vi "Interfaz grafica - corriente.vi"() -> ()   [LabVIEW 2024]
uses:
  160620 Optotune Lens Driver 4 Labview package/Hello Optotune Lens (30.06.2015)/Calibration.ctl
  <vilib>/Utility/file.llb/Read Delimited Spreadsheet (string).vi
  <vilib>/Instr/_visa.llb/VISA Configure Serial Port (Instr).vi
  <vilib>/Utility/file.llb/Write Delimited Spreadsheet (string).vi
panel:
  in  "Numeric WL control":i32
  in  "stop 6":bool
  in  "stop 5":bool
  in  "stop 4":bool
  in  "stop 3":bool
  in  "stop 2":bool
  in  "stop":bool
  out "Array 4":string[](array[string])
  out "Array 3":string[](array[string])
  out "Array 2":string[](array[string])
  out "Array":string[](array[string])
  out "Nombre 2":string
  in  "Restablecer Iniciales":bool
  in  "Incremento":dbl=0.1 format="%#_13g"
  out "Potencia derecho":dbl
  out "error out 4":errorcluster
  out "error out 3":errorcluster
  out "error out 2":errorcluster
  out "VISA resource name out":string
  in  "Tab Control 2":T1(tab)
  in  "Potencia inicial lente derecho":dbl(slide) scale=-3.0..3.0
  in  "Potencia inicial lente izquierdo":dbl(slide) scale=-3.0..3.0
  in  "VISA resource name":string="COM11"
  in  "VISA resource name 2":string="COM10"
  out "DPT INICIALES D":dbl
  out "DPT INICIALES I":dbl
  out "Potencia izquierdo":dbl
  in  "error in (no error) 5":errorcluster
  in  "error in (no error) 4":errorcluster
  in  "error in (no error) 3":errorcluster
  in  "error in (no error) 2":errorcluster
  in  "Calibration 4":T2={"Max Current A"=293.0, "Max Current B"=293.0, "UCL A"=300.0, "UCL B"=300.0, "LCL A"=0.0, "LCL B"=0.0} {"Max Current A" format="%#_g mA"; "Max Current B" format="%#_g mA"; "UCL A" format="%#_g mA"; "LCL A" format="%#_g mA"; "UCL B" format="%#_g mA"; "LCL B" format="%#_g mA"}
  out "ID 2":u16
  out "VISA resource name out 2":string
  out "Calibration 3":T2 {"Max Current A" format="%#_g mA"; "Max Current B" format="%#_g mA"; "UCL A" format="%#_g mA"; "LCL A" format="%#_g mA"; "UCL B" format="%#_g mA"; "LCL B" format="%#_g mA"}
  out "OK 2":bool
  out "Data 2":string
  out "Command to Port 2":string
  in  "Calibration":T2={"Max Current A"=293.0, "Max Current B"=293.0, "UCL A"=300.0, "UCL B"=300.0, "LCL A"=0.0, "LCL B"=0.0} {"Max Current A" format="%#_g mA"; "Max Current B" format="%#_g mA"; "UCL A" format="%#_g mA"; "LCL A" format="%#_g mA"; "UCL B" format="%#_g mA"; "LCL B" format="%#_g mA"}
  out "ID":u16
  out "Calibration 2":T2 {"Max Current A" format="%#_g mA"; "Max Current B" format="%#_g mA"; "UCL A" format="%#_g mA"; "LCL A" format="%#_g mA"; "UCL B" format="%#_g mA"; "LCL B" format="%#_g mA"}
  out "OK":bool
  out "Data":string
  out "Command to Port":string
  in  "DPT dif.":dbl
  out "error out":errorcluster
  in  "error in (no error)":errorcluster
  out "T button?":bool
  in  "Elegir menu Exp":bool
  in  "Elegir menu":bool
  out "path":path
  in  "Iniciar experimento":bool
  out "Enfermedad visual":string
  out "Edad":string
  out "Nombre":string
  out "Cedula":string
  in  "Carpeta":path=path "C:/Users/TGM1603/Documents/LabVIEW Data/Experimentos electrodos"
  in  "?":bool
  in  "Menu Principal":u16(ring) items=["Visualizacion general ", "Llevar a cabo un experimento", "Ajustar potencia inicial lentes"]
  in  "Menu experimentos":u16(ring) items=["Experimento 1", "Experimento 2", "Experimento 3", "Experimento 4"]
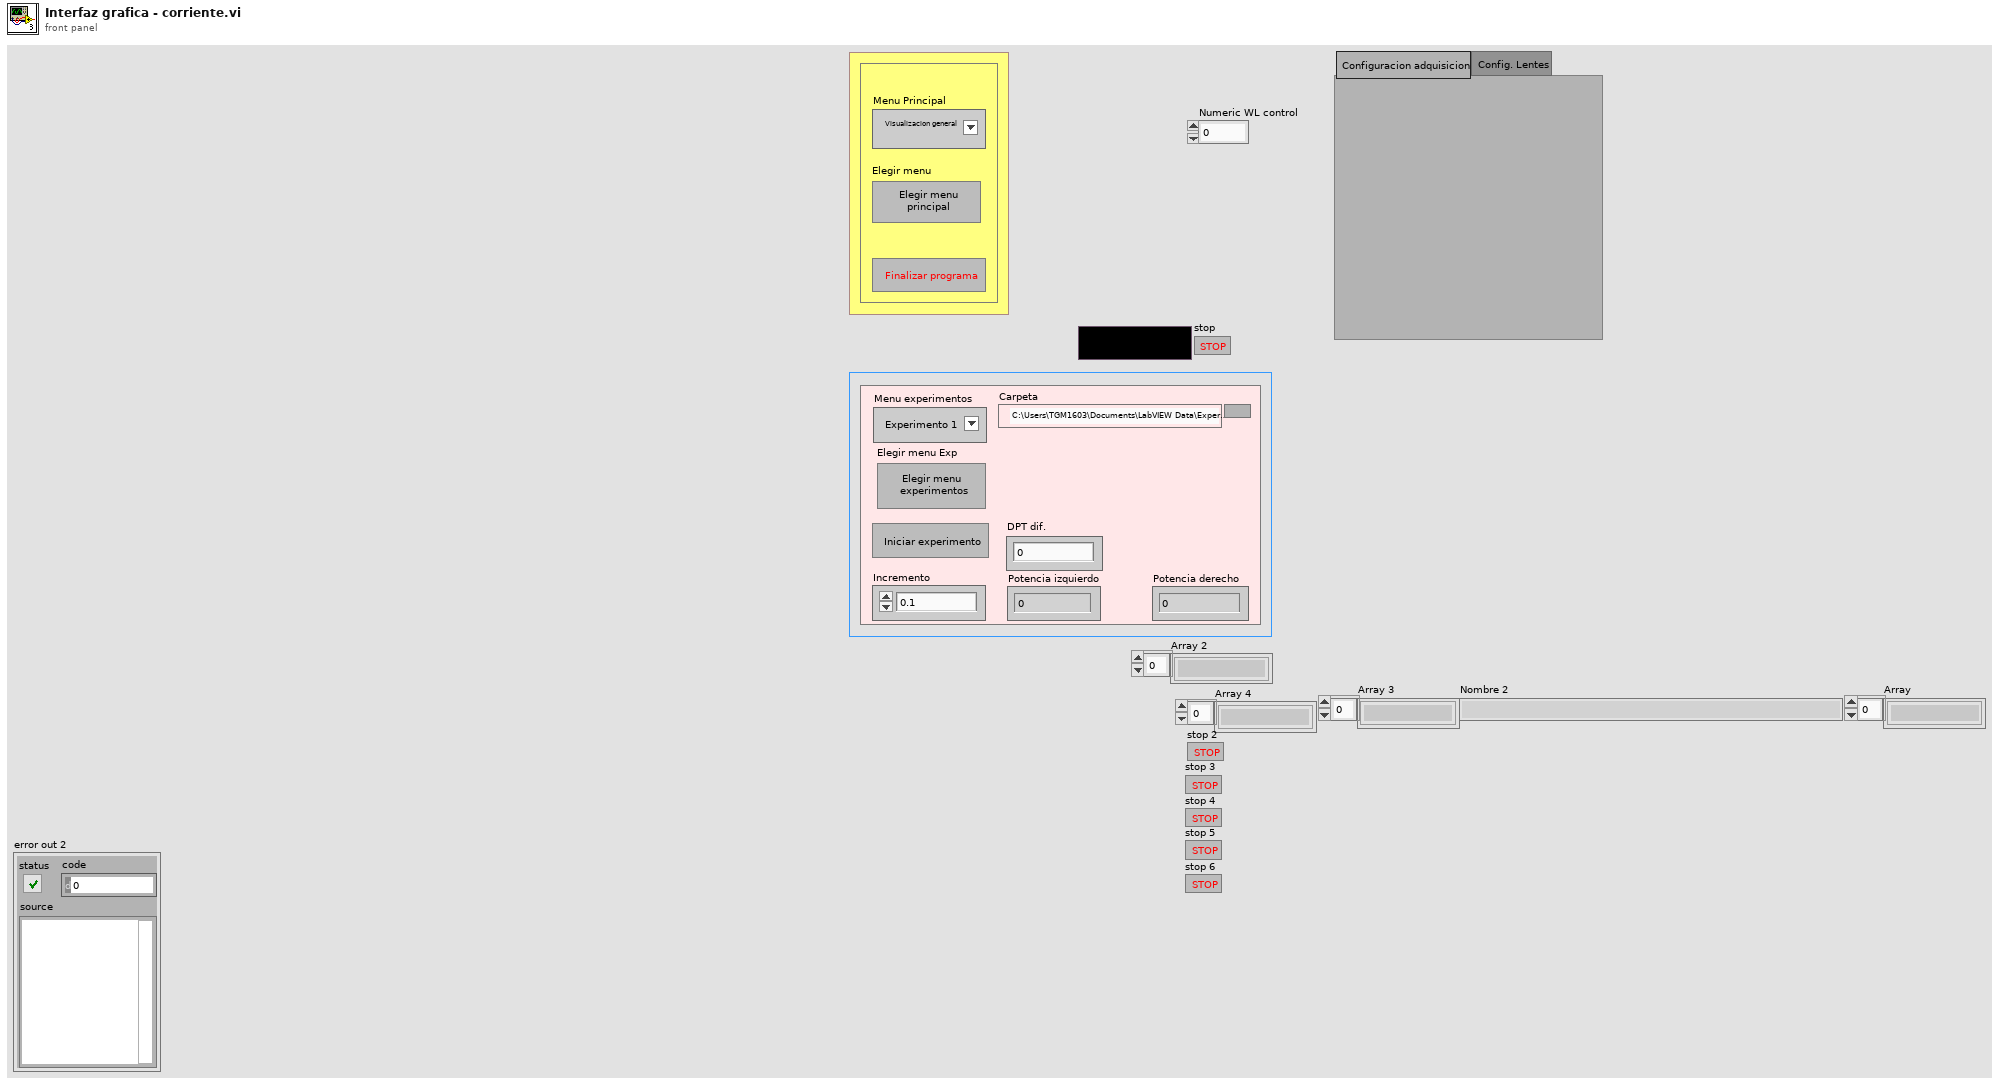
[diagram p1: front panel]
types:
  T1 = enum32{"Configuracion adquisicion", "Config. Lentes"}
  T2 = typedef "Calibration.ctl" = cluster{"Max Current A":dbl, "Max Current B":dbl, "UCL A":dbl, "UCL B":dbl, "LCL A":dbl, "LCL B":dbl}
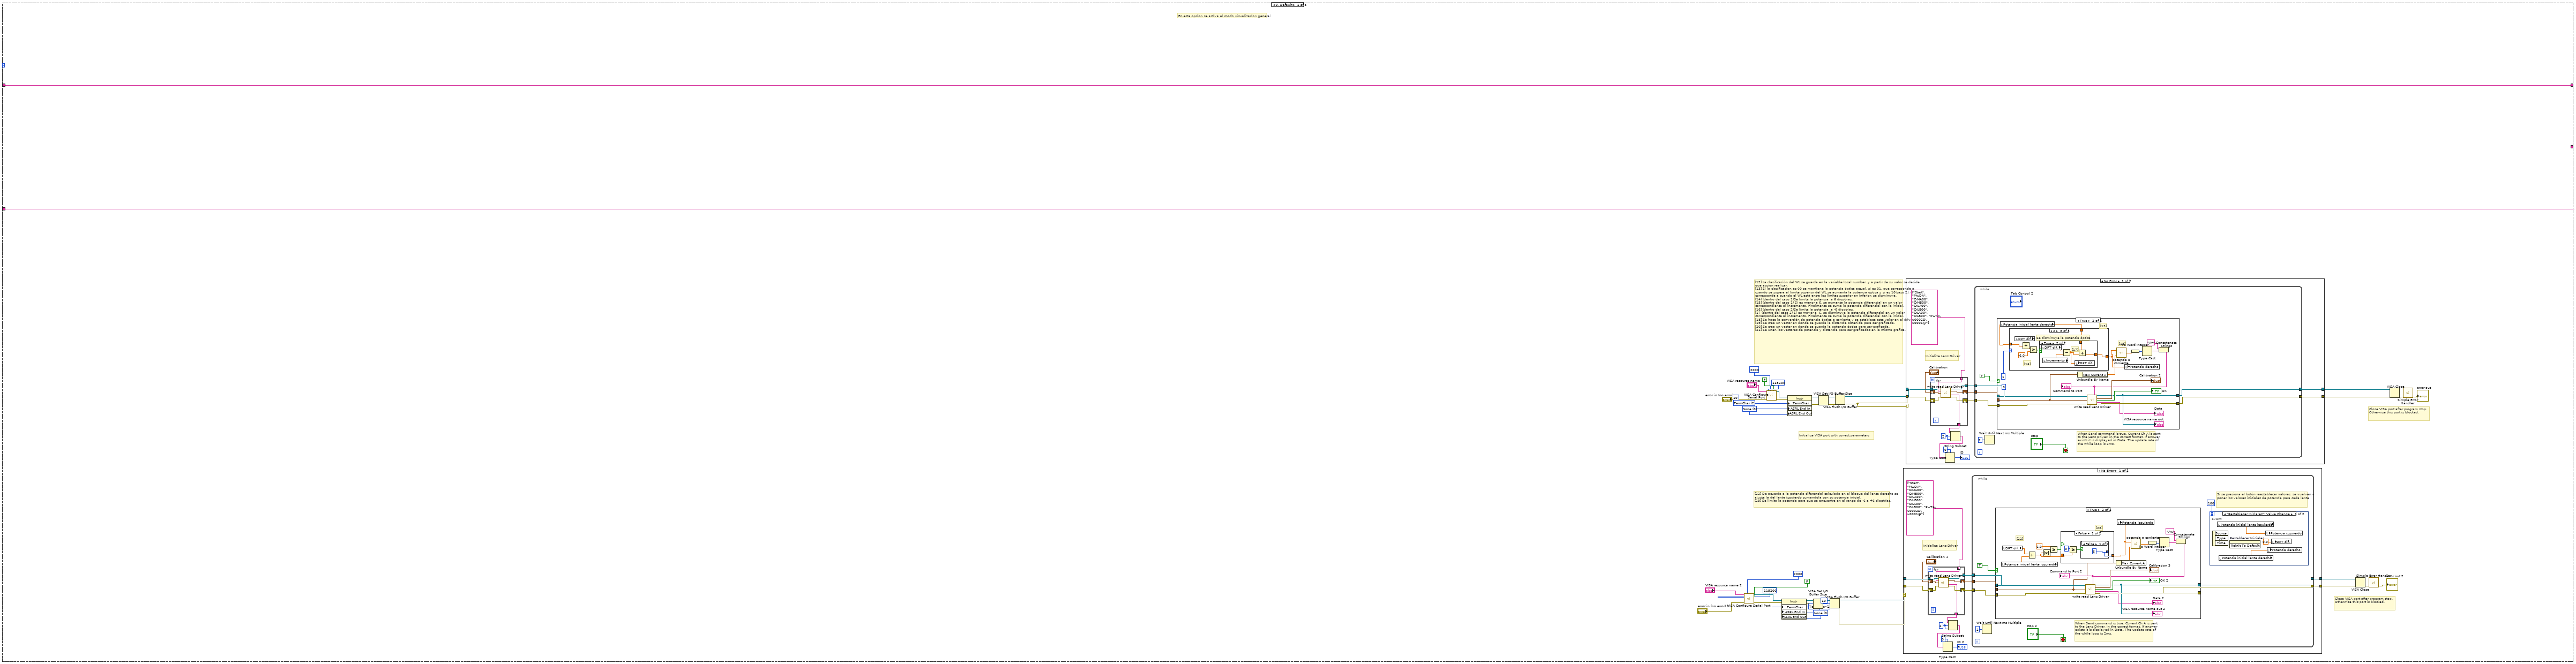
[diagram p2: hidden frame]
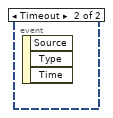
[diagram p3: hidden frame]
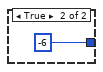
[diagram p5: hidden frame]
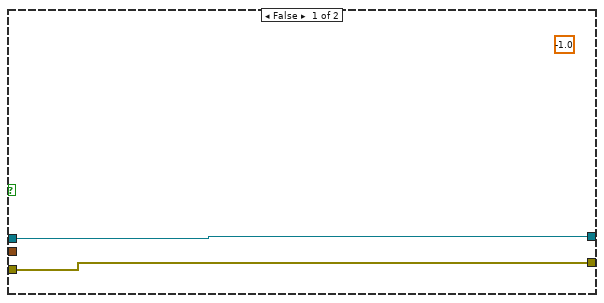
[diagram p8: hidden frame]
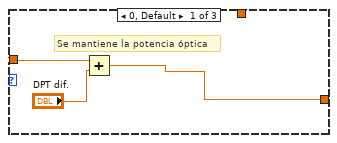
[diagram p9: hidden frame]
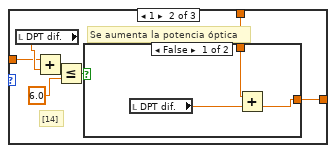
[diagram p10: hidden frame]
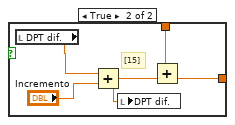
[diagram p11: hidden frame]
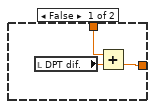
[diagram p12: hidden frame]
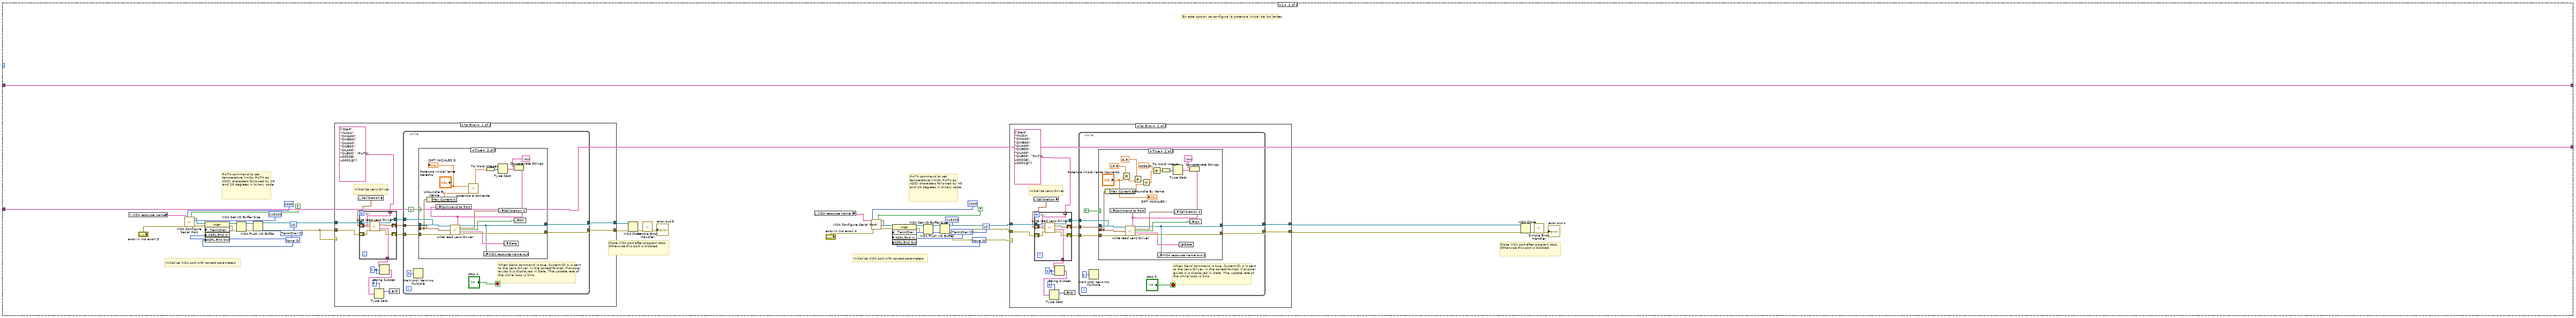
[diagram p14: hidden frame]
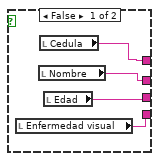
[diagram p19: hidden frame]
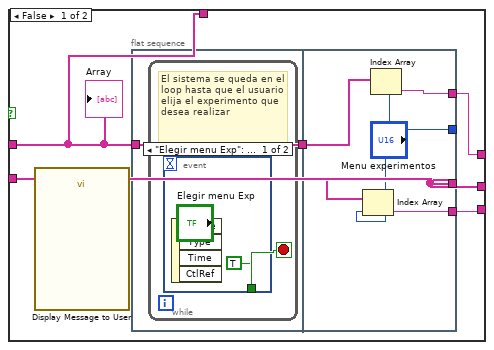
[diagram p20: hidden frame]
diagram:
  n1 = flat-sequence {
    tunnel: [w9] -> w2
    tunnel: [w6] -> w1
    tunnel: w2 -> [w13]
    tunnel: w1 -> [w14]
    frame #0 {
      # "Se inicializan los valores\nde potencia óptica y WL"
      # "Crea la cola que va a guardar los valores de la sumatoria que calcula el waveform length así como determina la cantidad de valores que se van a sumar(tamaño de la ventana)"
      # "Se obtiene los elementos de la columna 1 que corresponde a  la descripcion de los experimentos"
      # "Se obtiene los elementos de la columna 0 que corresponde al nombre de los experimentos"
      # "Se guarda los experimentos en el menu\n para que el usuario pueda elegir cual \nrealizar"
      # "Se cargan los experimentos  guardados"
      n2 = call-poly <vilib>:"Read Delimited Spreadsheet.vi"("file path (dialog if empty)"=path "C:/Users/willi/GITHUB/TG/Interfaz grafica -LabVIEW/Try 1/TG Juan Diego/Documentos de Labview/Experimentos_realizados") -> ("all rows"=w10:string[][])  [unwired: 9 in, 5 out]
      n3 = Transpose 2D Array(2D array=w10) -> (transposed array=w7:string[][])
      n4 = Index Array(array=w7, index (row)=1) -> (element=w6:string[])  [unwired: 1 in]
      n5 = Index Array(array=w7, index (row)=0) -> (element=w9:string[])  [unwired: 1 in]
      n6 = property on="Menu experimentos" class="Ring (strict)"("Strings []"=w9) -> ()  [unwired: 2 in, 2 out]
      n7 = local write "DPT INICIALES D"(0.0 ("DPT INIT.1")) -> ()
      n8 = local write "DPT INICIALES I"(0.0 ("DPT INIT.2")) -> ()
      n9 = local write "DPT dif."(0.0 ("WL")) -> ()
    }
    frame #1 {
      n10 = while {
        shift-right: [w19] -> _
        shift-left: w13 -> [w20]
        shift-right: [w17] -> _
        shift-left: w14 -> [w18]
        stop <- w16 stop-if-true
        n11 = event shown="[0] \"Elegir menu\": Value Change" {
          selector: _ -> [_ _]
          dyn-events: _ -> [_ _]
          timeout: 10 -> [_ _]
          tunnel: w20 -> [w25 w718]
          tunnel: [w24 w718] -> w19
          tunnel: w18 -> [w23 w717]
          tunnel: [w22 w717] -> w17
          tunnel: [_ "?"] -> w16
          event "Elegir menu": Value Change {
            n12 = event-data() -> ()  [unwired: 1 in, 6 out]
            n13 = case shown="1" "Menu Principal" {
              tunnel: w25 -> [w67 w259 w372]
              tunnel: [w67 w259 w371] -> w24
              tunnel: w23 -> [w66 w258 w369]
              tunnel: [w66 w258 w368] -> w22
              frame 0, Default {
                w41 = u16 0 items=["None", "Last Bit", "TermChar", "Break"] ("Serial Settings:End Mode for Writes")
                w40 = u16 2 items=["None", "Last Bit", "TermChar"] ("Serial Settings:End Mode for Reads")
                w56 = u16 0 items=["None", "Last Bit", "TermChar", "Break"] ("Serial Settings:End Mode for Writes")
                w57 = u16 2 items=["None", "Last Bit", "TermChar"] ("Serial Settings:End Mode for Reads")
                # "[22] De acuerda a la potencia diferencial calculada en el bloque del lente derecho se ajusta la del lente izquierdo sumandola con su potencia inicial.\n[23] Se limita la potencia para que se encuentre en el rango de -6 a +6 dioptrías."
                # "[12] La clasificación del WL se guarda en la variable local number, y a partir de su valor se decide que accion realizar.\n[13] Si la clasificacion es 00 se mantiene la potencia óptica actual, si es 01, que corresponde a cuando se supera el limite superior del WL,se aumenta la potencia óptica y si es 10(caso 2), que corresponde a cuando el WL está entre los limites superior en inferior, se disminuye. \n[14] (dentro del caso 1)Se limita la potencia  a 6 dioptrías. \n[15] (dentro del caso 1) Si es menor a 6, se aumenta la potencia diferencial en un valor correspondiente al incremento. Finalmente se suma la potencia diferencial con la inicial.\n[16] (dentro del caso 2)Se limita la potencia  a -6 dioptrías.\n[17 (dentro del caso 2) Si es mayor a -6, se disminuye la potencia diferencial en un valor correspondiente al incremento. Finalmente se suma la potencia diferencial con la inicial.\n[18] Se hace la conversión de potencia óptica a corriente y se establece este valor en el driver.\n[19] Se crea un vector en donde se guarda la distancia obtenida para ser graficada.\n[20] Se crea un vector en donde se guarda la potencia óptica para ser graficada.\n[21] Se unen los vectores de potencia y distancia para ser graficados en la misma grafica."
                # "En esta opcion se activa el modo visualizacion general"
                # "Close VISA port after program stop. Otherwise this port is blocked."
                # "Close VISA port after program stop. Otherwise this port is blocked."
                # "Initialize VISA port with correct parameters"
                n14 = call-poly "VISA Configure Serial Port"("VISA resource name"="VISA resource name 2", "timeout (10sec)"=u32 2000, "Enable Termination\nChar (T)"=FALSE ("Enable Termination\nChar (T)"), "baud rate (9600)"=u32 115200, "error in (no error)"="error in (no error) 2") -> ("VISA resource name out"=w36:refnum<visa-resource-name>, "error out"=w38:errorcluster)  [unwired: 9 in]
                n15 = call-poly "VISA Configure Serial Port"("VISA resource name"="VISA resource name", "timeout (10sec)"=u32 2000, "Enable Termination\nChar (T)"=FALSE ("Enable Termination\nChar (T)"), "baud rate (9600)"=u32 115200, "error in (no error)"="error in (no error)") -> ("VISA resource name out"=w61:refnum<visa-resource-name>, "error out"=w59:errorcluster)  [unwired: 9 in]
                n16 = property class="Instr"(reference=w36, error in=w38, "TermChar"=u8 10 ("Message Based Settings:Termination Character"), "ASRL End In"=w40, "ASRL End Out"=w41) -> (reference out=w37:refnum<visa-resource-name>, error out=w39:errorcluster)
                n17 = property class="Instr"(reference=w61, error in=w59, "TermChar"=u8 10 ("Message Based Settings:Termination Character"), "ASRL End In"=w57, "ASRL End Out"=w56) -> (reference out=w60:refnum<visa-resource-name>, error out=w58:errorcluster)
                n18 = VISA Set I/O Buffer Size(VISA resource name=w37, error in (no error)=w39) -> (VISA resource name out=w44:refnum<visa-resource-name>, error out=w45:errorcluster)  [unwired: 2 in]
                n19 = VISA Set I/O Buffer Size(VISA resource name=w60, error in (no error)=w58) -> (VISA resource name out=w53:refnum<visa-resource-name>, error out=w52:errorcluster)  [unwired: 2 in]
                n20 = VISA Flush I/O Buffer(VISA resource name=w44, error in (no error)=w45) -> (VISA resource name out=w30:refnum<visa-resource-name>, error out=w31:errorcluster)  [unwired: 1 in]
                n21 = VISA Flush I/O Buffer(VISA resource name=w53, error in (no error)=w52) -> (VISA resource name out=w51:refnum<visa-resource-name>, error out=w46:errorcluster)  [unwired: 1 in]
                n22 = case shown="No Error" w31 {
                  tunnel: w31 -> [w81 w132]
                  tunnel: w30 -> [w80 w133]
                  tunnel: [w79 w132] -> w26
                  tunnel: [w78 w133] -> w27
                  frame No Error {
                    w76 = 2 ("length (rest)")
                    # "Initialize Lens Driver"
                    n23 = for {
                      tunnel: w80 -> [w130]
                      tunnel: [w127] -> w70
                      tunnel: string[] ["Start", "MwDA", "CrMA00", "CrMB00", "CrUA00", "CrUB00", "CrLA00", "CrLB00", "PwTA\u0002Ð\u0001@"] -> [w125] mode=indexing
                      tunnel: [w124] -> w69
                      shift-right: [w128] -> w71
                      shift-left: "Calibration 4" -> [w129]
                      shift-right: [w126] -> w72
                      shift-left: w81 -> [w131]
                      n24 = call "write read Lens Driver.vi"("VISA resource name"=w130, "command"=w125, "Calibration"=w129, "error in (no error)"=w131) -> ("VISA resource name out"=w127:refnum<visa-resource-name>, "Calibration 2"=w128:T2, "Data"=w124:string, "error out"=w126:errorcluster)  [unwired: 4 in, 4 out]
                    }
                    n25 = String Subset(string=w69, offset (0)=w76, length (rest)=w76) -> (substring=w74:string)
                    n26 = Type Cast(type=u16 0 ("length (rest)"), x=w74) -> (*(type *) &x=→"ID 2":u16)
                    n27 = while {
                      tunnel: [w84] -> w79
                      tunnel: [w85] -> w78
                      tunnel: w72 -> [w90]
                      tunnel: w71 -> [w89]
                      tunnel: w70 -> [w88]
                      stop <- "stop 2" stop-if-true
                      # "Si se presiona el botón reestablecer valores, se vuelven a poner los valores iniciales de potencia para cada lente"
                      # "When Send command is true, Current Ch A is sent to the Lens Driver, in the correct format. If answer exists it is displayed in Data. The update rate of the while loop is 2ms."
                      n28 = Wait Until Next ms Multiple(millisecond multiple=u32 2) -> ()  [unwired: 1 out]
                      n29 = case shown="True" TRUE ("Send command") {
                        tunnel: [w95 w116] -> w84
                        tunnel: w90 -> [w95 w115]
                        tunnel: w89 -> [_ w97]
                        tunnel: w88 -> [w94 w114]
                        tunnel: [w94 w111] -> w85
                        frame False {
                        }
                        frame True {
                          # "[23]"
                          # "[22]"
                          n30 = local read "Potencia inicial lente izquierdo"() -> (w105:dbl)
                          n31 = local read "DPT dif."() -> (w106:dbl)
                          n32 = Add(x=w106, y=w105) -> (x+y=w101:dbl)
                          n33 = Absolute Value(x=w101) -> (abs(x)=w103:dbl)
                          n34 = Greater Or Equal?(x=6.0, y=w103) -> (x >= y?=w104:bool)
                          n35 = case shown="False" w104 {
                            tunnel: w101 -> [w119 w123]
                            tunnel: [w117 w123] -> w99
                            frame False {
                              n36 = Greater Or Equal?(x=u16 0, y=w119) -> (x >= y?=w120:bool)
                              n37 = case shown="False" w120 {
                                tunnel: [i16 6 ("x") i16 -6 ("x")] -> w117
                                frame False {
                                }
                                frame True {
                                }
                              }
                            }
                            frame True {
                            }
                          }
                          n38 = Unbundle By Name(w97) -> ("Max Current A"=w98:dbl)
                          n39 = local write "Potencia izquierdo"(w99) -> ()
                          n40 = call "potencia a corriente.vi"("Max current A"=w98, "Potencia"=w99) -> ("Corriente"=w100:dbl)
                          n41 = To Word Integer(number=w100) -> (16bit integer=w109:i16)
                          n42 = Type Cast(x=w109) -> (*(type *) &x=w108:string)  [unwired: 1 in]
                          n43 = Concatenate Strings("Aw", w108) -> (w107:string)
                          "Command to Port 2" <- w107
                          n44 = call "write read Lens Driver.vi"("VISA resource name"=w114, "command"=w107, "Calibration"=w97, "error in (no error)"=w115) -> ("VISA resource name out"=w111:refnum<visa-resource-name>, "Calibration 2"=→"Calibration 3":T2, "OK"=→"OK 2":bool, "Data"=→"Data 2":string, "error out"=w116:errorcluster)  [unwired: 4 in, 3 out]
                          "VISA resource name out 2" <- w111
                        }
                      }
                      n45 = event shown="[0] \"Restablecer Iniciales\": Value Change" {
                        selector: _ -> [_ _]
                        dyn-events: _ -> [_ _]
                        timeout: 100 -> [_ _]
                        event "Restablecer Iniciales": Value Change {
                          n46 = event-data() -> ()  [unwired: 1 in, 3 out]
                          n47 = local read "Potencia inicial lente izquierdo"() -> (w91:dbl)
                          n48 = local read "Potencia inicial lente derecho"() -> (w92:dbl)
                          n49 = invoke on="Restablecer Iniciales" class="Bool" method="Reinit To Default"() -> ()  [unwired: 3 in, 3 out]
                          n50 = local write "Potencia izquierdo"(w91) -> ()
                          n51 = local write "Potencia derecho"(w92) -> ()
                          n52 = local write "DPT dif."(0.0 ("DPT dif.")) -> ()
                        }
                        event Timeout {
                          n53 = event-data() -> ()  [unwired: 1 in, 3 out]
                        }
                      }
                    }
                  }
                  frame Error {
                  }
                }
                n54 = case shown="No Error" w46 {
                  tunnel: w46 -> [w147 w216]
                  tunnel: w51 -> [w146 w217]
                  tunnel: [w145 w216] -> w49
                  tunnel: [w144 w217] -> w47
                  frame No Error {
                    w142 = 2 ("length (rest)")
                    # "Initialize Lens Driver"
                    n55 = for {
                      tunnel: w146 -> [w214]
                      tunnel: [w211] -> w136
                      tunnel: string[] ["Start", "MwDA", "CrMA00", "CrMB00", "CrUA00", "CrUB00", "CrLA00", "CrLB00", "PwTA\u0002Ð\u0001@"] -> [w209] mode=indexing
                      tunnel: [w208] -> w135
                      shift-right: [w212] -> w137
                      shift-left: "Calibration" -> [w213]
                      shift-right: [w210] -> w138
                      shift-left: w147 -> [w215]
                      n56 = call "write read Lens Driver.vi"("VISA resource name"=w214, "command"=w209, "Calibration"=w213, "error in (no error)"=w215) -> ("VISA resource name out"=w211:refnum<visa-resource-name>, "Calibration 2"=w212:T2, "Data"=w208:string, "error out"=w210:errorcluster)  [unwired: 4 in, 4 out]
                    }
                    n57 = String Subset(string=w135, offset (0)=w142, length (rest)=w142) -> (substring=w140:string)
                    n58 = Type Cast(type=u16 0 ("length (rest)"), x=w140) -> (*(type *) &x=→"ID":u16)
                    n59 = while {
                      tunnel: [w149] -> w145
                      tunnel: [w150] -> w144
                      tunnel: w138 -> [w155]
                      tunnel: w137 -> [w154]
                      tunnel: w136 -> [w153]
                      stop <- "stop" stop-if-true
                      # "When Send command is true, Current Ch A is sent to the Lens Driver, in the correct format. If answer exists it is displayed in Data. The update rate of the while loop is 2ms."
                      n60 = Wait Until Next ms Multiple(millisecond multiple=u32 2) -> ()  [unwired: 1 out]
                      n61 = case shown="True" TRUE ("Send command") {
                        tunnel: [w157 w174] -> w149
                        tunnel: w155 -> [w157 w173]
                        tunnel: w154 -> [_ w161]
                        tunnel: w153 -> [w156 w172]
                        tunnel: [w156 w169] -> w150
                        frame False {
                          (unwired) -1.0 ("DPT")
                        }
                        frame True {
                          (unwired) 0
                          # "[18]"
                          # "[13]"
                          n62 = local read "Potencia inicial lente derecho"() -> (w164:dbl)
                          n63 = case shown="2" 1 {
                            tunnel: [w176 w184 w199] -> w163
                            tunnel: w164 -> [w177 w179 w194]
                            tunnel: w164 -> [_ w178 w193]
                            frame 0, Default {
                              # "Se mantiene la potencia óptica"
                              n64 = Add(x=w177, y="DPT dif.") -> (x+y=w176:dbl)
                            }
                            frame 1 {
                              # "[14]"
                              # "Se aumenta la potencia óptica"
                              n65 = local read "DPT dif."() -> (w180:dbl)
                              n66 = Add(x=w179, y=w180) -> (x+y=w181:dbl)
                              n67 = Less Or Equal?(x=w181, y=6.0) -> (x <= y?=w183:bool)
                              n68 = case shown="False" w183 {
                                tunnel: [w186 w189] -> w184
                                tunnel: w178 -> [w185 w188]
                                frame False {
                                n69 = local read "DPT dif."() -> (w187:dbl)
                                n70 = Add(x=w185, y=w187) -> (x+y=w186:dbl)
                                }
                                frame True {
                                # "[15]"
                                n71 = local read "DPT dif."() -> (w190:dbl)
                                n72 = Add(x=w190, y="Incremento") -> (x+y=w191:dbl)
                                n73 = local write "DPT dif."(w191) -> ()
                                n74 = Add(x=w188, y=w191) -> (x+y=w189:dbl)
                                }
                              }
                            }
                            frame 2 {
                              # "[16]"
                              # "Se disminuye la potencia óptica"
                              n75 = local read "DPT dif."() -> (w198:dbl)
                              n76 = Add(x=w198, y=w194) -> (x+y=w195:dbl)
                              n77 = Greater Or Equal?(x=w195, y=-6.0) -> (x >= y?=w196:bool)
                              n78 = case shown="True" w196 {
                                tunnel: [w201 w205] -> w199
                                tunnel: w193 -> [w200 w204]
                                frame False {
                                n79 = local read "DPT dif."() -> (w202:dbl)
                                n80 = Add(x=w200, y=w202) -> (x+y=w201:dbl)
                                }
                                frame True {
                                # "[17]"
                                n81 = local read "DPT dif."() -> (w207:dbl)
                                n82 = local read "Incremento"() -> (w203:dbl)
                                n83 = Subtract(x=w207, y=w203) -> (x-y=w206:dbl)
                                n84 = local write "DPT dif."(w206) -> ()
                                n85 = Add(x=w204, y=w206) -> (x+y=w205:dbl)
                                }
                              }
                            }
                          }
                          n86 = Unbundle By Name(w161) -> ("Max Current A"=w160:dbl)
                          n87 = call "potencia a corriente.vi"("Max current A"=w160, "Potencia"=w163) -> ("Corriente"=w162:dbl)
                          n88 = local write "Potencia derecho"(w163) -> ()
                          n89 = To Word Integer(number=w162) -> (16bit integer=w167:i16)
                          n90 = Type Cast(x=w167) -> (*(type *) &x=w166:string)  [unwired: 1 in]
                          n91 = Concatenate Strings("Aw", w166) -> (w165:string)
                          "Command to Port" <- w165
                          n92 = call "write read Lens Driver.vi"("VISA resource name"=w172, "command"=w165, "Calibration"=w161, "error in (no error)"=w173) -> ("VISA resource name out"=w169:refnum<visa-resource-name>, "Calibration 2"=→"Calibration 2":T2, "OK"=→"OK":bool, "Data"=→"Data":string, "error out"=w174:errorcluster)  [unwired: 4 in, 3 out]
                          "VISA resource name out" <- w169
                        }
                      }
                    }
                  }
                  frame Error {
                  }
                }
                n93 = VISA Close(VISA resource name=w27, error in (no error)=w26) -> (error out=w28:errorcluster)
                n94 = call <vilib>:"Simple Error Handler.vi"("error in (no error)"=w28) -> ("error out"=→"error out 2":errorcluster)  [unwired: 4 in, 4 out]
                n95 = VISA Close(VISA resource name=w47, error in (no error)=w49) -> (error out=w50:errorcluster)
                n96 = call <vilib>:"Simple Error Handler.vi"("error in (no error)"=w50) -> ("error out"=→"error out":errorcluster)  [unwired: 4 in, 4 out]
              }
              frame 2 {
                w238 = u16 0 items=["None", "Last Bit", "TermChar", "Break"] ("Serial Settings:End Mode for Writes")
                w237 = u16 2 items=["None", "Last Bit", "TermChar"] ("Serial Settings:End Mode for Reads")
                w251 = u16 0 items=["None", "Last Bit", "TermChar", "Break"] ("Serial Settings:End Mode for Writes")
                w250 = u16 2 items=["None", "Last Bit", "TermChar"] ("Serial Settings:End Mode for Reads")
                # "En esta opcion se configura la potencia inicial de los lentes"
                # "Close VISA port after program stop. Otherwise this port is blocked."
                # "Close VISA port after program stop. Otherwise this port is blocked."
                # "PwTA command to set temperature limits: PwTA as ASCII characters followed by 45 and 20 degrees in binary code."
                # "Initialize VISA port with correct parameters"
                # "PwTA command to set temperature limits: PwTA as ASCII characters followed by 45 and 20 degrees in binary code."
                # "Initialize VISA port with correct parameters"
                n97 = local read "VISA resource name"() -> (w228:string)
                n98 = call-poly "VISA Configure Serial Port"("VISA resource name"=w228, "timeout (10sec)"=u32 2000, "Enable Termination\nChar (T)"=FALSE ("Enable Termination\nChar (T)"), "baud rate (9600)"=u32 115200, "error in (no error)"="error in (no error) 3") -> ("VISA resource name out"=w233:refnum<visa-resource-name>, "error out"=w235:errorcluster)  [unwired: 9 in]
                n99 = property class="Instr"(reference=w233, error in=w235, "TermChar"=u8 10 ("Message Based Settings:Termination Character"), "ASRL End In"=w237, "ASRL End Out"=w238) -> (reference out=w234:refnum<visa-resource-name>, error out=w236:errorcluster)
                n100 = VISA Set I/O Buffer Size(VISA resource name=w234, error in (no error)=w236) -> (VISA resource name out=w240:refnum<visa-resource-name>, error out=w241:errorcluster)  [unwired: 2 in]
                n101 = VISA Flush I/O Buffer(VISA resource name=w240, error in (no error)=w241) -> (VISA resource name out=w227:refnum<visa-resource-name>, error out=w226:errorcluster)  [unwired: 1 in]
                n102 = case shown="No Error" w226 {
                  tunnel: w226 -> [w273 w307]
                  tunnel: w227 -> [w272 w308]
                  tunnel: [w271 w307] -> w222
                  tunnel: [w270 w308] -> w223
                  frame No Error {
                    w269 = 2 ("length (rest)")
                    # "Initialize Lens Driver"
                    n103 = local read "Calibration"() -> (w261:T2)
                    n104 = for {
                      tunnel: w272 -> [w305]
                      tunnel: [w302] -> w264
                      tunnel: string[] ["Start", "MwDA", "CrMA00", "CrMB00", "CrUA00", "CrUB00", "CrLA00", "CrLB00", "PwTA\u0002Ð\u0001@"] -> [w300] mode=indexing
                      tunnel: [w299] -> w263
                      shift-right: [w303] -> w265
                      shift-left: w261 -> [w304]
                      shift-right: [w301] -> w266
                      shift-left: w273 -> [w306]
                      n105 = call "write read Lens Driver.vi"("VISA resource name"=w305, "command"=w300, "Calibration"=w304, "error in (no error)"=w306) -> ("VISA resource name out"=w302:refnum<visa-resource-name>, "Calibration 2"=w303:T2, "Data"=w299:string, "error out"=w301:errorcluster)  [unwired: 4 in, 4 out]
                    }
                    n106 = String Subset(string=w263, offset (0)=w269, length (rest)=w269) -> (substring=w267:string)
                    n107 = Type Cast(type=u16 0 ("length (rest)"), x=w267) -> (*(type *) &x=w262:u16)
                    n108 = local write "ID"(w262) -> ()
                    n109 = while {
                      tunnel: [w275] -> w271
                      tunnel: [w276] -> w270
                      tunnel: w266 -> [w281]
                      tunnel: w265 -> [w280]
                      tunnel: w264 -> [w279]
                      stop <- "stop 4" stop-if-true
                      # "When Send command is true, Current Ch A is sent to the Lens Driver, in the correct format. If answer exists it is displayed in Data. The update rate of the while loop is 2ms."
                      n110 = Wait Until Next ms Multiple(millisecond multiple=u32 2) -> ()  [unwired: 1 out]
                      n111 = case shown="True" TRUE ("Send command") {
                        tunnel: [w283 w298] -> w275
                        tunnel: w281 -> [w283 w297]
                        tunnel: w280 -> [_ w288]
                        tunnel: w279 -> [w282 w296]
                        tunnel: [w282 w289] -> w276
                        frame False {
                        }
                        frame True {
                          n112 = Unbundle By Name(w288) -> ("Max Current A"=w287:dbl)
                          n113 = call "potencia a corriente.vi"("Max current A"=w287, "Potencia"="Potencia inicial lente derecho") -> ("Corriente"=w285:dbl)
                          n114 = To Word Integer(number=w285) -> (16bit integer=w295:i16)
                          n115 = Type Cast(x=w295) -> (*(type *) &x=w294:string)  [unwired: 1 in]
                          n116 = Concatenate Strings("Aw", w294) -> (w291:string)
                          n117 = local write "Command to Port"(w291) -> ()
                          n118 = call "write read Lens Driver.vi"("VISA resource name"=w296, "command"=w291, "Calibration"=w288, "error in (no error)"=w297) -> ("VISA resource name out"=w289:refnum<visa-resource-name>, "Calibration 2"=w293:T2, "OK"=w292:bool, "Data"=w290:string, "error out"=w298:errorcluster)  [unwired: 4 in, 3 out]
                          n119 = local write "VISA resource name out"(w289) -> ()
                          n120 = local write "Calibration 2"(w293) -> ()
                          n121 = local write "Data"(w290) -> ()
                          n122 = local write "OK"(w292) -> ()
                          "DPT INICIALES D" <- "Potencia inicial lente derecho"
                        }
                      }
                    }
                  }
                  frame Error {
                  }
                }
                n123 = VISA Close(VISA resource name=w223, error in (no error)=w222) -> (error out=w225:errorcluster)
                n124 = call <vilib>:"Simple Error Handler.vi"("error in (no error)"=w225) -> ("error out"=→"error out 3":errorcluster)  [unwired: 4 in, 4 out]
                n125 = local read "VISA resource name 2"() -> (w242:string)
                n126 = call-poly "VISA Configure Serial Port"("VISA resource name"=w242, "timeout (10sec)"=u32 2000, "Enable Termination\nChar (T)"=FALSE ("Enable Termination\nChar (T)"), "baud rate (9600)"=u32 115200, "error in (no error)"="error in (no error) 4") -> ("VISA resource name out"=w246:refnum<visa-resource-name>, "error out"=w248:errorcluster)  [unwired: 9 in]
                n127 = property class="Instr"(reference=w246, error in=w248, "TermChar"=u8 10 ("Message Based Settings:Termination Character"), "ASRL End In"=w250, "ASRL End Out"=w251) -> (reference out=w247:refnum<visa-resource-name>, error out=w249:errorcluster)
                n128 = VISA Set I/O Buffer Size(VISA resource name=w247, error in (no error)=w249) -> (VISA resource name out=w253:refnum<visa-resource-name>, error out=w254:errorcluster)  [unwired: 2 in]
                n129 = VISA Flush I/O Buffer(VISA resource name=w253, error in (no error)=w254) -> (VISA resource name out=w256:refnum<visa-resource-name>, error out=w255:errorcluster)  [unwired: 1 in]
                n130 = case shown="No Error" w255 {
                  tunnel: w255 -> [w322 w362]
                  tunnel: w256 -> [w321 w363]
                  tunnel: [w320 w362] -> w219
                  tunnel: [w319 w363] -> w218
                  frame No Error {
                    w318 = 2 ("length (rest)")
                    # "Initialize Lens Driver"
                    n131 = local read "Calibration"() -> (w310:T2)
                    n132 = for {
                      tunnel: w321 -> [w360]
                      tunnel: [w357] -> w313
                      tunnel: string[] ["Start", "MwDA", "CrMA00", "CrMB00", "CrUA00", "CrUB00", "CrLA00", "CrLB00", "PwTA\u0002Ð\u0001@"] -> [w355] mode=indexing
                      tunnel: [w354] -> w312
                      shift-right: [w358] -> w314
                      shift-left: w310 -> [w359]
                      shift-right: [w356] -> w315
                      shift-left: w322 -> [w361]
                      n133 = call "write read Lens Driver.vi"("VISA resource name"=w360, "command"=w355, "Calibration"=w359, "error in (no error)"=w361) -> ("VISA resource name out"=w357:refnum<visa-resource-name>, "Calibration 2"=w358:T2, "Data"=w354:string, "error out"=w356:errorcluster)  [unwired: 4 in, 4 out]
                    }
                    n134 = String Subset(string=w312, offset (0)=w318, length (rest)=w318) -> (substring=w316:string)
                    n135 = Type Cast(type=u16 0 ("length (rest)"), x=w316) -> (*(type *) &x=w311:u16)
                    n136 = local write "ID"(w311) -> ()
                    n137 = while {
                      tunnel: [w324] -> w320
                      tunnel: [w325] -> w319
                      tunnel: w315 -> [w330]
                      tunnel: w314 -> [w329]
                      tunnel: w313 -> [w328]
                      stop <- "stop 3" stop-if-true
                      # "When Send command is true, Current Ch A is sent to the Lens Driver, in the correct format. If answer exists it is displayed in Data. The update rate of the while loop is 2ms."
                      n138 = Wait Until Next ms Multiple(millisecond multiple=u32 2) -> ()  [unwired: 1 out]
                      n139 = case shown="True" TRUE ("Send command") {
                        tunnel: [w332 w353] -> w324
                        tunnel: w330 -> [w332 w352]
                        tunnel: w329 -> [_ w340]
                        tunnel: w328 -> [w331 w351]
                        tunnel: [w331 w341] -> w325
                        frame False {
                        }
                        frame True {
                          n140 = Unbundle By Name(w340) -> ("Max Current A"=w339:dbl)
                          n141 = Multiply(x=15.8, y="Potencia inicial lente izquierdo") -> (x*y=w337:dbl)
                          n142 = Add(x=-6.8, y=w337) -> (x+y=w335:dbl)
                          n143 = Divide(x=w335, y=w339) -> (x/y=w338:dbl)
                          n144 = Multiply(x=4096.0, y=w338) -> (x*y=w349:dbl)
                          n145 = To Word Integer(number=w349) -> (16bit integer=w348:i16)
                          n146 = Type Cast(x=w348) -> (*(type *) &x=w347:string)  [unwired: 1 in]
                          n147 = Concatenate Strings("Aw", w347) -> (w343:string)
                          n148 = local write "Command to Port"(w343) -> ()
                          n149 = call "write read Lens Driver.vi"("VISA resource name"=w351, "command"=w343, "Calibration"=w340, "error in (no error)"=w352) -> ("VISA resource name out"=w341:refnum<visa-resource-name>, "Calibration 2"=w345:T2, "OK"=w344:bool, "Data"=w342:string, "error out"=w353:errorcluster)  [unwired: 4 in, 3 out]
                          n150 = local write "VISA resource name out 2"(w341) -> ()
                          n151 = local write "Calibration 2"(w345) -> ()
                          n152 = local write "Data"(w342) -> ()
                          n153 = local write "OK"(w344) -> ()
                          "DPT INICIALES I" <- "Potencia inicial lente izquierdo"
                        }
                      }
                    }
                  }
                  frame Error {
                  }
                }
                n154 = VISA Close(VISA resource name=w218, error in (no error)=w219) -> (error out=w221:errorcluster)
                n155 = call <vilib>:"Simple Error Handler.vi"("error in (no error)"=w221) -> ("error out"=→"error out 4":errorcluster)  [unwired: 4 in, 4 out]
              }
              frame 1 {
                (unwired) dbl[][] [[0.0]] ("History Data")
                (unwired) dbl[][] [[0.0]] ("History Data")
                # "Mensaje que pregunta si desea realizar el experimento\ncon un nuevo usuario o con el actual"
                # "Se vuelven 0 los valores del WL y de la potencia óptica y distancia"
                # "En esta opcion se activa el modo experimento"
                n156 = Two Button Dialog(message="Con quien desea realizar los experimentos?", 1:"Nuevo voluntario" ("F button name (\"Cancel\")"), 2:"Voluntario actual" ("T button name (\"OK\")")) -> (T button?=w375:bool)
                n157 = flat-sequence {
                  tunnel: w375 -> [w387]
                  tunnel: [w386] -> w373
                  tunnel: w372 -> [w386]
                  tunnel: [w396] -> w376
                  tunnel: [w398] -> w374
                  tunnel: w373 -> [w398]
                  tunnel: [w397] -> w370
                  tunnel: w369 -> [w397]
                  tunnel: w376 -> [w409]
                  tunnel: w374 -> [w408]
                  tunnel: [w407] -> w371
                  tunnel: w370 -> [w406]
                  tunnel: [w405] -> w367
                  tunnel: [w404] -> w366
                  tunnel: [w403] -> w364
                  tunnel: w367 -> [w452]
                  tunnel: w366 -> [w435]
                  tunnel: [w452] -> w365
                  tunnel: w364 -> [w438]
                  tunnel: [w454] -> w368
                  tunnel: w365 -> [w454]
                  frame #0 {
                    # "Se guardan los datos de un nuevo voluntario"
                    n158 = Not(x=w387) -> (.not. x?=w381:bool)
                    n159 = case shown="True" w381 {
                      tunnel: [w390 w395] -> w385
                      tunnel: [w389 w394] -> w384
                      tunnel: [w391 w393] -> w383
                      tunnel: [w388 w392] -> w382
                      frame False {
                        n160 = local read "Enfermedad visual"() -> (w390:string)
                        n161 = local read "Nombre"() -> (w391:string)
                        n162 = local read "Cedula"() -> (w388:string)
                        n163 = local read "Edad"() -> (w389:string)
                      }
                      frame True {
                        n164 = call "Registro voluntario"() -> ("Enfermedad visual"=w395:string, "Edad"=w394:string, "Cedula"=w392:string, "Nombre"=w393:string)  [unwired: 14 in, 2 out]
                      }
                    }
                    "Cedula" <- w382
                    "Nombre" <- w383
                    "Edad" <- w384
                    "Enfermedad visual" <- w385
                    n165 = local write "T button?"(FALSE ("T button?")) -> ()
                  }
                  frame #1 {
                    n166 = Two Button Dialog(message="Qué tipo de experimento desea realizar?", 1:"Nuevo Experimento" ("F button name (\"Cancel\")"), 2:"Experimento existente" ("T button name (\"OK\")")) -> (T button?=w399:bool)
                    n167 = Not(x=w399) -> (.not. x?=w396:bool)
                  }
                  frame #2 {
                    # "A partir de la seleccion del experimento, se obtiene la descripcion correspondiente que será guardada en el archivo"
                    n168 = case shown="True" w409 {
                      tunnel: w408 -> [w411 w429]
                      tunnel: [w411 w428] -> w407
                      tunnel: w406 -> [w413 w427]
                      tunnel: [w413 w426] -> w405
                      tunnel: [w414 w425] -> w404
                      tunnel: [w410 w424] -> w403
                      frame False {
                        n169 = call "Display Message to User"() -> ()  [unwired: 10 in, 2 out]
                        n170 = flat-sequence {
                          tunnel: [w415] -> w412
                          tunnel: w411 -> [w415]
                          tunnel: [w423] -> w414
                          tunnel: w413 -> [w422]
                          tunnel: ["Menu experimentos"] -> _
                          tunnel: w412 -> [w420]
                          tunnel: [w419] -> w410
                          frame #0 {
                            n171 = while {
                              stop <- w416 stop-if-true
                              # "El sistema se queda en el loop hasta que el usuario elija el experimento que desea realizar"
                              n172 = event shown="[0] \"Elegir menu Exp\": Value Change" {
                                selector: _ -> [_ _]
                                dyn-events: _ -> [_ _]
                                timeout: _ -> [_ _]
                                tunnel: [TRUE FALSE] -> w416
                                event "Elegir menu Exp": Value Change {
                                n173 = event-data() -> ()  [unwired: 1 in, 4 out]
                                }
                                event Timeout {
                                n174 = event-data() -> ()  [unwired: 1 in, 3 out]
                                }
                              }
                            }
                          }
                          frame #1 {
                            n175 = Index Array(array=w422, index="Menu experimentos") -> (element=w423:string)
                            n176 = Index Array(array=w420, index="Menu experimentos") -> (element=w419:string)
                          }
                        }
                        "Array" <- w411
                      }
                      frame True {
                        # "Se añade el nuevo experimento al menu de seleccion de experimentos"
                        # "Se guarda el nuevo experimento en el archivo que los contiene"
                        n177 = call "Nuevo experimento"() -> ("Descripcion"=w425:string, "Nombre"=w424:string)  [unwired: 16 in, 2 out]
                        n178 = Insert Into Array(array=w427, new element=w425) -> (w426:string[])  [unwired: 1 in]
                        n179 = Insert Into Array(array=w429, new element=w424) -> (w428:string[])  [unwired: 1 in]
                        n180 = property on="Menu experimentos" class="Ring (strict)"("Strings []"=w428) -> ()  [unwired: 2 in, 2 out]
                        n181 = Insert Into Array(array=string[] [], new element #1=w424, new element #2=w425) -> (w431:string[])  [unwired: 1 in]
                        n182 = call-poly <vilib>:"Write Delimited Spreadsheet.vi"("file path (dialog if empty)"=path "C:/Users/willi/GITHUB/TG/Interfaz grafica -LabVIEW/Try 1/TG Juan Diego/Documentos de Labview/Experimentos_realizados", "1D data"=w431, "append to file? (new file:F)"=TRUE) -> ()  [unwired: 11 in, 2 out]
                      }
                    }
                  }
                  frame #3 {
                    # "Se guardan los datos generales del experimento en el archivo de excel"
                    n183 = local read "Enfermedad visual"() -> (w437:string)
                    n184 = local read "Cedula"() -> (w439:string)
                    n185 = local read "Edad"() -> (w436:string)
                    n186 = local read "Nombre"() -> (w440:string)
                    n187 = Get Date/Time In Seconds() -> (seconds since 1Jan1904=w451:timestamp)
                    n188 = Format Date/Time String(time format string (%c)="_%d-%m-%y_%H-%M", seconds (now)=w451) -> (date/time string=w449:string)  [unwired: 1 in]
                    n189 = Path To String(path="Carpeta") -> (string=w447:string)
                    n190 = local read "Cedula"() -> (w443:string)
                    n191 = call "MS Office Report"("Path to Save Report"=path "C:/Users/willi/GITHUB/TG/Interfaz grafica -LabVIEW/Try 1/TG Juan Diego/Documentos de Labview/save_report_TRY1.xlsx", "Cedula"=w439, "Edad"=w436, "Enfermedad"=w437, "Exp_nombre"=w438, "Experimento"=w435, "Nombre"=w440) -> ()  [unwired: 19 in, 2 out]
                    n192 = Concatenate Strings(w447, "\\" ("string"), w443, w449, "_" ("string"), w438, ".xlsx" ("string")) -> (w445:string)
                    n193 = String To Path(string=w445) -> (path=→"path":path)
                    "Nombre 2" <- w438
                  }
                  frame #4 {
                    n194 = while {
                      shift-right: [w455] -> _
                      shift-left: enum16{"Inicio", "Tomar datos", ""}."Inicio" -> [w457]
                      stop <- w456 stop-if-true
                      n195 = case shown="\"Tomar datos\"" w457 {
                        tunnel: [w458 w464] -> w455
                        frame "Inicio", Default {
                          # "Se chequea si el usuario ha presionado el boton de comenzar el experimento. Si no lo ha hecho, se queda en este estado (0).\n Cuando lo presiona, pasa al estado de adquirir datios (1) ."
                          n196 = Select(t=enum16{"Inicio", "Tomar datos", ""}."Tomar datos", s="Iniciar experimento", f=enum16{"Inicio", "Tomar datos", ""}."Inicio") -> (s? t:f=w458:enum16{"Inicio", "Tomar datos", ""})
                        }
                        frame "Tomar datos" {
                          n197 = flat-sequence {
                            tunnel: [w515] -> w463
                            tunnel: [w497] -> w462
                            tunnel: w463 -> [w709]
                            tunnel: w462 -> [w710]
                            tunnel: [enum16{"Inicio", "Tomar datos", ""}."Inicio"] -> w464
                            frame #0 {
                              w487 = u16 0 items=["None", "Last Bit", "TermChar", "Break"] ("Serial Settings:End Mode for Writes")
                              w488 = u16 2 items=["None", "Last Bit", "TermChar"] ("Serial Settings:End Mode for Reads")
                              w506 = u16 0 items=["None", "Last Bit", "TermChar", "Break"] ("Serial Settings:End Mode for Writes")
                              w507 = u16 2 items=["None", "Last Bit", "TermChar"] ("Serial Settings:End Mode for Reads")
                              # "[9] Se unen en una sola matriz los vectores de tiempo, distancia, potencia derecha y potencia izquierda."
                              # "[9]"
                              # "[8]"
                              # "[7]"
                              # "[6]"
                              # "[5]"
                              # "Se usan registros de desplazamiento para concatenar en un solo vector los datos que se obtienen en cada iteracion. Así en \n[1] Se guarda la potencia del lente derecho.\n[2] Por medio de variables locales, se guarda la distancia que se obtuvo en el bloque de distancia.\n[3]  Por medio de variables locales, se guarda la potencia del lente izquierdo que se obtuvo en el bloque de control de potencia del lente izquierdo.\n[4] Se guarda el tiempo actual.\n[5] Se pasa el vector de de potencia derecha a variable a string con 2 cifras significativas. \n[6] Se ajusta el vector del tiempo para que se muestre un tiempo relativo, es decir, en donde el primer dato sea 0 y en los demas se aumente un dt.  Además, se pasa el vector a variable a string con 5 cifras significativas.\n[7] Se pasa el vector de de distancia a variable a string con 0 cifras significativas. \n[8] Se pasa el vector de de potencia izquierda a variable a string con 2 cifras significativas."
                              # "Initialize VISA port with correct parameters"
                              # "Initialize VISA port with correct parameters"
                              # "Close VISA port after program stop. Otherwise this port is blocked."
                              # "[12]"
                              n198 = local read "error in (no error)"() -> (w502:errorcluster)
                              n199 = local read "VISA resource name"() -> (w501:string)
                              n200 = local read "VISA resource name 2"() -> (w483:string)
                              n201 = call-poly "VISA Configure Serial Port"("VISA resource name"=w501, "timeout (10sec)"=u32 2000, "Enable Termination\nChar (T)"=FALSE ("Enable Termination\nChar (T)"), "baud rate (9600)"=u32 115200, "error in (no error)"=w502) -> ("VISA resource name out"=w511:refnum<visa-resource-name>, "error out"=w509:errorcluster)  [unwired: 9 in]
                              n202 = call-poly "VISA Configure Serial Port"("VISA resource name"=w483, "timeout (10sec)"=u32 2000, "Enable Termination\nChar (T)"=FALSE ("Enable Termination\nChar (T)"), "baud rate (9600)"=u32 115200, "error in (no error)"="error in (no error) 5") -> ("VISA resource name out"=w492:refnum<visa-resource-name>, "error out"=w490:errorcluster)  [unwired: 9 in]
                              n203 = property class="Instr"(reference=w511, error in=w509, "TermChar"=u8 10 ("Message Based Settings:Termination Character"), "ASRL End In"=w507, "ASRL End Out"=w506) -> (reference out=w510:refnum<visa-resource-name>, error out=w508:errorcluster)
                              n204 = property class="Instr"(reference=w492, error in=w490, "TermChar"=u8 10 ("Message Based Settings:Termination Character"), "ASRL End In"=w488, "ASRL End Out"=w487) -> (reference out=w491:refnum<visa-resource-name>, error out=w489:errorcluster)
                              n205 = VISA Set I/O Buffer Size(VISA resource name=w510, error in (no error)=w508) -> (VISA resource name out=w504:refnum<visa-resource-name>, error out=w503:errorcluster)  [unwired: 2 in]
                              n206 = VISA Set I/O Buffer Size(VISA resource name=w491, error in (no error)=w489) -> (VISA resource name out=w485:refnum<visa-resource-name>, error out=w484:errorcluster)  [unwired: 2 in]
                              n207 = VISA Flush I/O Buffer(VISA resource name=w504, error in (no error)=w503) -> (VISA resource name out=w500:refnum<visa-resource-name>, error out=w499:errorcluster)  [unwired: 1 in]
                              n208 = VISA Flush I/O Buffer(VISA resource name=w485, error in (no error)=w484) -> (VISA resource name out=w481:refnum<visa-resource-name>, error out=w480:errorcluster)  [unwired: 1 in]
                              n209 = case shown="No Error" w480 {
                                tunnel: w480 -> [w543 w600]
                                tunnel: w481 -> [w542 w601]
                                tunnel: [w541 w600] -> w469
                                tunnel: [w540 w601] -> w468
                                tunnel: [w530 dbl[] [-30.0]] -> _
                                frame No Error {
                                w539 = 2 ("length (rest)")
                                # "Bloque de control del izquierdo. Se explica en el caso 0 de visualziación general"
                                # "Initialize Lens Driver"
                                n210 = local read "Calibration"() -> (w531:T2)
                                n211 = for {
                                tunnel: w542 -> [w597]
                                tunnel: [w594] -> w534
                                tunnel: string[] ["Start", "MwDA", "CrMA00", "CrMB00", "CrUA00", "CrUB00", "CrLA00", "CrLB00", "PwTA\u0002Ð\u0001@"] -> [w592] mode=indexing
                                tunnel: [w591] -> w533
                                shift-right: [w595] -> w535
                                shift-left: w531 -> [w596]
                                shift-right: [w593] -> w536
                                shift-left: w543 -> [w598]
                                n212 = call "write read Lens Driver.vi"("VISA resource name"=w597, "command"=w592, "Calibration"=w596, "error in (no error)"=w598) -> ("VISA resource name out"=w594:refnum<visa-resource-name>, "Calibration 2"=w595:T2, "Data"=w591:string, "error out"=w593:errorcluster)  [unwired: 4 in, 4 out]
                                }
                                n213 = String Subset(string=w533, offset (0)=w539, length (rest)=w539) -> (substring=w537:string)
                                n214 = Type Cast(type=u16 0 ("length (rest)"), x=w537) -> (*(type *) &x=w532:u16)
                                n215 = local write "ID"(w532) -> ()
                                n216 = while {
                                tunnel: [w548] -> w541
                                tunnel: [w549] -> w540
                                tunnel: w536 -> [w554]
                                tunnel: w535 -> [w553]
                                tunnel: w534 -> [w552]
                                shift-right: [w546] -> w530
                                shift-left: _ -> [w547]
                                stop <- "stop 6" stop-if-true
                                # "When Send command is true, Current Ch A is sent to the Lens Driver, in the correct format. If answer exists it is displayed in Data. The update rate of the while loop is 2ms."
                                n217 = case shown="True" TRUE ("Send command") {
                                tunnel: [w560 w583] -> w548
                                tunnel: w554 -> [w560 w582]
                                tunnel: w553 -> [_ w563]
                                tunnel: w552 -> [w559 w581]
                                tunnel: [w559 w574] -> w549
                                tunnel: [dbl[] [-20.0] w573] -> w546
                                tunnel: w547 -> [_ w572]
                                frame False {
                                }
                                frame True {
                                n218 = local read "Potencia inicial lente izquierdo"() -> (w571:dbl)
                                n219 = local read "DPT dif."() -> (w570:dbl)
                                n220 = Add(x=w570, y=w571) -> (x+y=w566:dbl)
                                n221 = Absolute Value(x=w566) -> (abs(x)=w568:dbl)
                                n222 = Greater Or Equal?(x=6.0, y=w568) -> (x >= y?=w567:bool)
                                n223 = case shown="True" w567 {
                                tunnel: w566 -> [w586 w590]
                                tunnel: [w584 w590] -> w564
                                frame False {
                                n224 = Greater Or Equal?(x=u16 0, y=w586) -> (x >= y?=w587:bool)
                                n225 = case shown="False" w587 {
                                tunnel: [i16 6 ("x") i16 -6 ("x")] -> w584
                                frame False {
                                }
                                frame True {
                                }
                                }
                                }
                                frame True {
                                }
                                }
                                "Potencia izquierdo" <- w564
                                n226 = Unbundle By Name(w563) -> ("Max Current A"=w562:dbl)
                                n227 = call "potencia a corriente.vi"("Max current A"=w562, "Potencia"=w564) -> ("Corriente"=w565:dbl)
                                n228 = To Word Integer(number=w565) -> (16bit integer=w580:i16)
                                n229 = Type Cast(x=w580) -> (*(type *) &x=w579:string)  [unwired: 1 in]
                                n230 = Concatenate Strings("Aw", w579) -> (w576:string)
                                n231 = local write "Command to Port"(w576) -> ()
                                n232 = call "write read Lens Driver.vi"("VISA resource name"=w581, "command"=w576, "Calibration"=w563, "error in (no error)"=w582) -> ("VISA resource name out"=w574:refnum<visa-resource-name>, "Calibration 2"=w578:T2, "OK"=w577:bool, "Data"=w575:string, "error out"=w583:errorcluster)  [unwired: 4 in, 3 out]
                                n233 = local write "VISA resource name 2"(w574) -> ()
                                n234 = local write "Calibration 2"(w578) -> ()
                                n235 = local write "Data"(w575) -> ()
                                n236 = local write "OK"(w577) -> ()
                                n237 = Build Array (concatenate)(w572, w564) -> (w573:dbl[])
                                }
                                }
                                n238 = Wait Until Next ms Multiple(millisecond multiple=u32 10) -> ()  [unwired: 1 out]
                                n239 = event shown="[0] \"Restablecer Iniciales\": Value Change" {
                                selector: _ -> [_ _]
                                dyn-events: _ -> [_ _]
                                timeout: 100 -> [_ _]
                                event "Restablecer Iniciales": Value Change {
                                n240 = event-data() -> ()  [unwired: 1 in, 3 out]
                                n241 = local read "Potencia inicial lente izquierdo"() -> (w555:dbl)
                                n242 = local read "Potencia inicial lente derecho"() -> (w556:dbl)
                                n243 = local write "Potencia izquierdo"(w555) -> ()
                                n244 = local write "Potencia derecho"(w556) -> ()
                                n245 = local write "DPT dif."(0.0 ("DPT dif.")) -> ()
                                }
                                event Timeout {
                                n246 = event-data() -> ()  [unwired: 1 in, 3 out]
                                }
                                }
                                }
                                }
                                frame Error {
                                }
                              }
                              n247 = case shown="No Error" w499 {
                                tunnel: w499 -> [w621 w705]
                                tunnel: w500 -> [w620 w706]
                                tunnel: [w619 w705] -> w527
                                tunnel: [w618 w706] -> w526
                                tunnel: [w607 dbl[] [-1.0]] -> w519
                                tunnel: [w606 dbl[] [-30.0]] -> w473
                                tunnel: [w604 dbl[] [-30.0]] -> w476
                                frame No Error {
                                w617 = 2 ("length (rest)")
                                # "Bloque de control del lente derecho. Se explica en el caso 0 de visualziación general"
                                # "Initialize Lens Driver"
                                n248 = local read "Calibration"() -> (w609:T2)
                                n249 = for {
                                tunnel: w620 -> [w700]
                                tunnel: [w697] -> w612
                                tunnel: string[] ["Start", "MwDA", "CrMA00", "CrMB00", "CrUA00", "CrUB00", "CrLA00", "CrLB00", "PwTA\u0002Ð\u0001@"] -> [w695] mode=indexing
                                tunnel: [w694] -> w611
                                shift-right: [w698] -> w613
                                shift-left: w609 -> [w699]
                                shift-right: [w696] -> w614
                                shift-left: w621 -> [w701]
                                n250 = call "write read Lens Driver.vi"("VISA resource name"=w700, "command"=w695, "Calibration"=w699, "error in (no error)"=w701) -> ("VISA resource name out"=w697:refnum<visa-resource-name>, "Calibration 2"=w698:T2, "Data"=w694:string, "error out"=w696:errorcluster)  [unwired: 4 in, 4 out]
                                }
                                n251 = String Subset(string=w611, offset (0)=w617, length (rest)=w617) -> (substring=w615:string)
                                n252 = Type Cast(type=u16 0 ("length (rest)"), x=w615) -> (*(type *) &x=w610:u16)
                                n253 = local write "ID"(w610) -> ()
                                n254 = while {
                                tunnel: [w632] -> w619
                                tunnel: [w633] -> w618
                                tunnel: w614 -> [w638]
                                tunnel: w613 -> [w637]
                                tunnel: w612 -> [w636]
                                shift-right: [w627] -> w607
                                shift-left: dbl[] [0.0] -> [w628]
                                shift-right: [w630] -> w606
                                shift-left: dbl[] [0.0] -> [w631]
                                shift-right: [w625] -> w604
                                shift-left: dbl[] [0.0] -> [w624]
                                stop <- "stop 5" stop-if-true
                                # "[4]"
                                # "[3]"
                                n255 = Wait Until Next ms Multiple(millisecond multiple=u32 10) -> ()  [unwired: 1 out]
                                n256 = case shown="True" TRUE ("Send command") {
                                tunnel: [w641 w660] -> w632
                                tunnel: w638 -> [w641 w659]
                                tunnel: w637 -> [_ w645]
                                tunnel: w636 -> [w640 w658]
                                tunnel: [w640 w651] -> w633
                                tunnel: [dbl[] [-20.0] w650] -> w630
                                tunnel: w631 -> [_ w649]
                                frame False {
                                }
                                frame True {
                                (unwired) 1
                                # "[1]"
                                n257 = local read "Potencia inicial lente derecho"() -> (w648:dbl)
                                n258 = case shown="1" "Numeric WL control" {
                                tunnel: [w661 w670 w685] -> w647
                                tunnel: w648 -> [w663 w665 w680]
                                tunnel: w648 -> [_ w664 w679]
                                frame 0, Default {
                                n259 = local read "DPT dif."() -> (w662:dbl)
                                n260 = Add(x=w663, y=w662) -> (x+y=w661:dbl)
                                }
                                frame 1 {
                                n261 = local read "DPT dif."() -> (w666:dbl)
                                n262 = Add(x=w665, y=w666) -> (x+y=w667:dbl)
                                n263 = Less Or Equal?(x=w667, y=6.0) -> (x <= y?=w669:bool)
                                n264 = case shown="True" w669 {
                                tunnel: [w672 w676] -> w670
                                tunnel: w664 -> [w671 w675]
                                frame False {
                                n265 = local read "DPT dif."() -> (w673:dbl)
                                n266 = Add(x=w671, y=w673) -> (x+y=w672:dbl)
                                }
                                frame True {
                                n267 = local read "DPT dif."() -> (w677:dbl)
                                n268 = local read "Incremento"() -> (w674:dbl)
                                n269 = Add(x=w677, y=w674) -> (x+y=w678:dbl)
                                n270 = local write "DPT dif."(w678) -> ()
                                n271 = Add(x=w675, y=w678) -> (x+y=w676:dbl)
                                }
                                }
                                }
                                frame 2 {
                                n272 = local read "DPT dif."() -> (w684:dbl)
                                n273 = Add(x=w684, y=w680) -> (x+y=w681:dbl)
                                n274 = Greater Or Equal?(x=w681, y=-6.0) -> (x >= y?=w682:bool)
                                n275 = case shown="True" w682 {
                                tunnel: [w687 w691] -> w685
                                tunnel: w679 -> [w686 w690]
                                frame False {
                                n276 = local read "DPT dif."() -> (w688:dbl)
                                n277 = Add(x=w686, y=w688) -> (x+y=w687:dbl)
                                }
                                frame True {
                                n278 = local read "DPT dif."() -> (w693:dbl)
                                n279 = local read "Incremento"() -> (w689:dbl)
                                n280 = Subtract(x=w693, y=w689) -> (x-y=w692:dbl)
                                n281 = local write "DPT dif."(w692) -> ()
                                n282 = Add(x=w690, y=w692) -> (x+y=w691:dbl)
                                }
                                }
                                }
                                }
                                "Potencia derecho" <- w647
                                n283 = Unbundle By Name(w645) -> ("Max Current A"=w644:dbl)
                                n284 = call "potencia a corriente.vi"("Max current A"=w644, "Potencia"=w647) -> ("Corriente"=w646:dbl)
                                n285 = To Word Integer(number=w646) -> (16bit integer=w657:i16)
                                n286 = Type Cast(x=w657) -> (*(type *) &x=w656:string)  [unwired: 1 in]
                                n287 = Concatenate Strings("Aw", w656) -> (w653:string)
                                n288 = local write "Command to Port"(w653) -> ()
                                n289 = call "write read Lens Driver.vi"("VISA resource name"=w658, "command"=w653, "Calibration"=w645, "error in (no error)"=w659) -> ("VISA resource name out"=w651:refnum<visa-resource-name>, "Calibration 2"=w655:T2, "OK"=w654:bool, "Data"=w652:string, "error out"=w660:errorcluster)  [unwired: 4 in, 3 out]
                                n290 = local write "VISA resource name out"(w651) -> ()
                                n291 = local write "Calibration 2"(w655) -> ()
                                n292 = local write "Data"(w652) -> ()
                                n293 = local write "OK"(w654) -> ()
                                n294 = Build Array (concatenate)(w649, w647) -> (w650:dbl[])
                                }
                                }
                                n295 = local read "Potencia izquierdo"() -> (w623:dbl)
                                n296 = Get Date/Time In Seconds() -> (seconds since 1Jan1904=w629:timestamp)
                                n297 = To Double Precision Float(number=w629) -> (double precision float=w626:dbl)
                                n298 = Build Array (concatenate)(w628, w626) -> (w627:dbl[])
                                n299 = Build Array (concatenate)(w624, w623) -> (w625:dbl[])
                                }
                                }
                                frame Error {
                                }
                              }
                              n300 = Delete From Array(array=w473, index=0) -> (array with subset deleted=w472:dbl[])  [unwired: 1 in, 1 out]
                              n301 = Index Array(array=w519, index=1) -> (element=w524:dbl)
                              n302 = Delete From Array(array=w476, index=0) -> (array with subset deleted=w475:dbl[])  [unwired: 1 in, 1 out]
                              n303 = VISA Close(VISA resource name=w468, error in (no error)=w469) -> (error out=w467:errorcluster)
                              n304 = Subtract(x=w519, y=w524) -> (x-y=w518:dbl[])
                              n305 = Number To Fractional String(use system decimal point (T)=FALSE, number=w472, precision (6)=i16 2) -> (F-format string=w496:string[])  [unwired: 1 in]
                              n306 = VISA Close(VISA resource name=w526, error in (no error)=w527) -> (error out=w528:errorcluster)
                              n307 = call <vilib>:"Simple Error Handler.vi"("error in (no error)"=w467) -> ("error out"=w466:errorcluster)  [unwired: 4 in, 4 out]
                              n308 = Delete From Array(array=w518, index=0) -> (array with subset deleted=w523:dbl[])  [unwired: 1 in, 1 out]
                              n309 = call <vilib>:"Simple Error Handler.vi"("error in (no error)"=w528) -> ("error out"=w525:errorcluster)  [unwired: 4 in, 4 out]
                              n310 = Number To Fractional String(use system decimal point (T)=FALSE, number=w475, precision (6)=i16 2) -> (F-format string=w477:string[])  [unwired: 1 in]
                              n311 = Number To Fractional String(use system decimal point (T)=FALSE, number=w523, precision (6)=i16 5) -> (F-format string=w465:string[])  [unwired: 1 in]
                              n312 = Build Array(w465, w496, w477) -> (w470:string[][])
                              n313 = Transpose 2D Array(2D array=w470) -> (transposed array=w497:string[][])
                              n314 = local write "error out"(w525) -> ()
                              n315 = local write "error out"(w466) -> ()
                              n316 = Build Array(w465, w496, w477) -> (w515:string[][])
                            }
                            frame #1 {
                              # "[13] En esta case structure, se decide que datos se van a guardar. Esto lo hace el SUBVI llamado guardar datos de amplitud y tiempo."
                              n317 = Transpose 2D Array(2D array=w709) -> ()  [unwired: 1 out]
                              n318 = call "Guardar datos de Amplitud y Tiempo.vi"("path"=path "C:/Users/willi/GITHUB/TG/Interfaz grafica -LabVIEW/Try 1/TG Juan Diego/Documentos de Labview/save_report_TRY1.xlsx", "Datos experimento"=w710, "column headers"=string[] ["Tiempo(s)", "Amplitud(V)"]) -> ()  [unwired: 3 in]
                            }
                            frame #2 {
                              # "Si el usuario desea repetir el experimento se vuelve al estado inicio en donde se espera que comience el experimento. De lo contrario se sale del loop y vuelve al menu principal."
                              n319 = Two Button Dialog(message="¿Desea repetir el experimento?", 1:"No" ("F button name (\"Cancel\")"), 2:"Si" ("T button name (\"OK\")")) -> (T button?=w713:bool)
                              n320 = Not(x=w713) -> (.not. x?=→"T button?":bool)
                            }
                          }
                        }
                      }
                      n321 = local read "T button?"() -> (w456:bool)
                    }
                  }
                }
                "Array 2" <- w372
              }
            }
          }
          event Timeout {
            n322 = event-data() -> ()  [unwired: 1 in, 3 out]
          }
        }
        "Array 3" <- w20
      }
      "Array 4" <- w13
    }
  }
